vi "CRYFrequency Shift.vi"(6 "User Sampling Rate":dbl, 7 "Freq Sampling Mode":i32, 9 "Reference Frequency":dbl, 10 "Source Wave Name":string, 11 "Waveform In":T1={"Waveform"={"X0"=0.0, "dX"=0.0, "Y"=array[57657 elements]}, "X data"=1, "Y data"=0, "Y axis"=0, "X unit"="s", "Y unit"="", "Y dB ref"=1.0, "display Y"=TRUE, "display X"=FALSE, "Overload?"=FALSE, "Test Info"="", "Step No."=0, "Name"="", "protected"=FALSE, "Sqc history"=[], "Signal Channel ID"=0, "Plot Settings"={"Color"=0, "Interpolation"=0, "Point Style"=0, "Line Style"=0, "Point Color"=0, "Line Width"=0, "Bar Plot Style"=0, "Fill To"=0}, "AutoProtect"=FALSE} {"Y dB ref" format="%.1f"; "Y axis" items=["Log", "Lin"]; "Y data" items=["dB", "Lin"]; "X data" items=["dB", "Lin"]}) -> (2 "PlaybackSamplingRate":dbl, 3 "Wave Out":T1={"Waveform"={"X0"=0.0, "dX"=0.0, "Y"=[]}, "X data"=1, "Y data"=1, "Y axis"=1, "X unit"="s", "Y unit"="V", "Y dB ref"=1.0, "display Y"=TRUE, "display X"=TRUE, "Overload?"=FALSE, "Test Info"="", "Step No."=0, "Name"="", "protected"=FALSE, "Sqc history"=[], "Signal Channel ID"=0, "Plot Settings"={"Color"=0, "Interpolation"=0, "Point Style"=0, "Line Style"=0, "Point Color"=0, "Line Width"=0, "Bar Plot Style"=0, "Fill To"=0}, "AutoProtect"=FALSE} {"Y dB ref" format="%.1f"; "Y axis" items=["Log", "Lin"]; "Y data" items=["dB", "Lin"]; "X data" items=["dB", "Lin"]})   [LabVIEW 2013]
uses:
  Typedef Control/CRYWaveform Cluster.ctl
  <vilib>/Analysis/3filter.llb/Filter Passband Type.ctl
  <vilib>/Analysis/4window.llb/windowTd.ctl
  <vilib>/Analysis/2dsp.llb/Real FFT.vi
  <vilib>/Analysis/3filter.llb/FIR Windowed Filter (DBL).vi
  <vilib>/Analysis/NI_AALPro.lvlib
  <vilib>/Analysis/NI_AALBase.lvlib
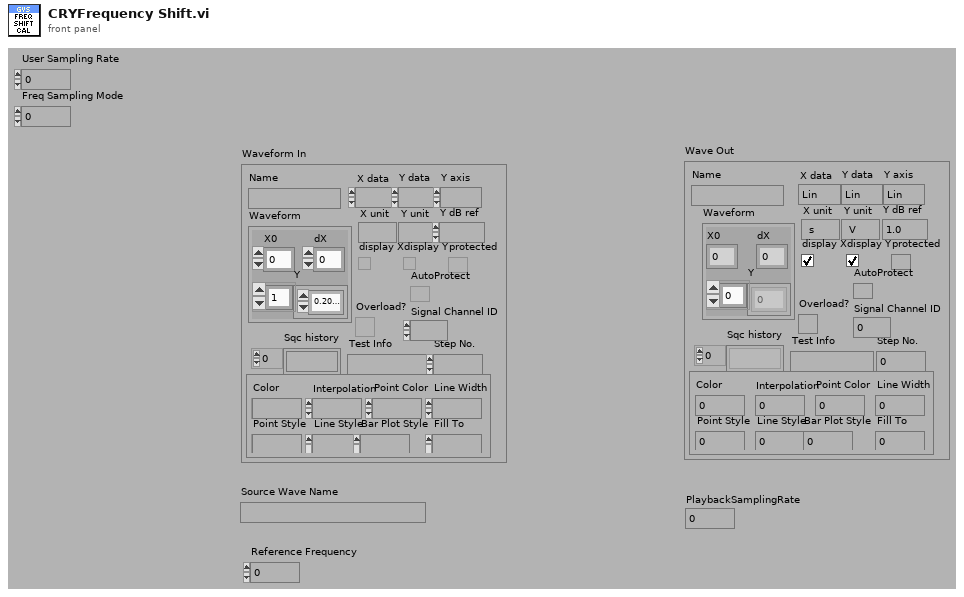
[diagram p1: front panel]
types:
  T1 = typedef "CRYWaveform Cluster.ctl" = cluster{"Waveform":cluster{"X0":dbl, "dX":dbl, "Y":sgl[]}, "X data":u16, "Y data":u16, "Y axis":u16, "X unit":string, "Y unit":string, "Y dB ref":dbl, "display Y":bool, "display X":bool, "Overload?":bool, "Test Info":string, "Step No.":i32, "Name":string, "protected":bool, "Sqc history":string[], "Signal Channel ID":i32, "Plot Settings":cluster{"Color":u32, "Interpolation":u8, "Point Style":u8, "Line Style":u8, "Point Color":u32, "Line Width":u8, "Bar Plot Style":u8, "Fill To":i16}, "AutoProtect":bool}
  T2 = typedef "NI_AALBase.lvlib/Filter Passband Type.ctl" = enum32{"Lowpass", "Highpass", "Bandpass", "Bandstop"}
  T3 = typedef "NI_AALPro.lvlib/windowTd.ctl" = u32
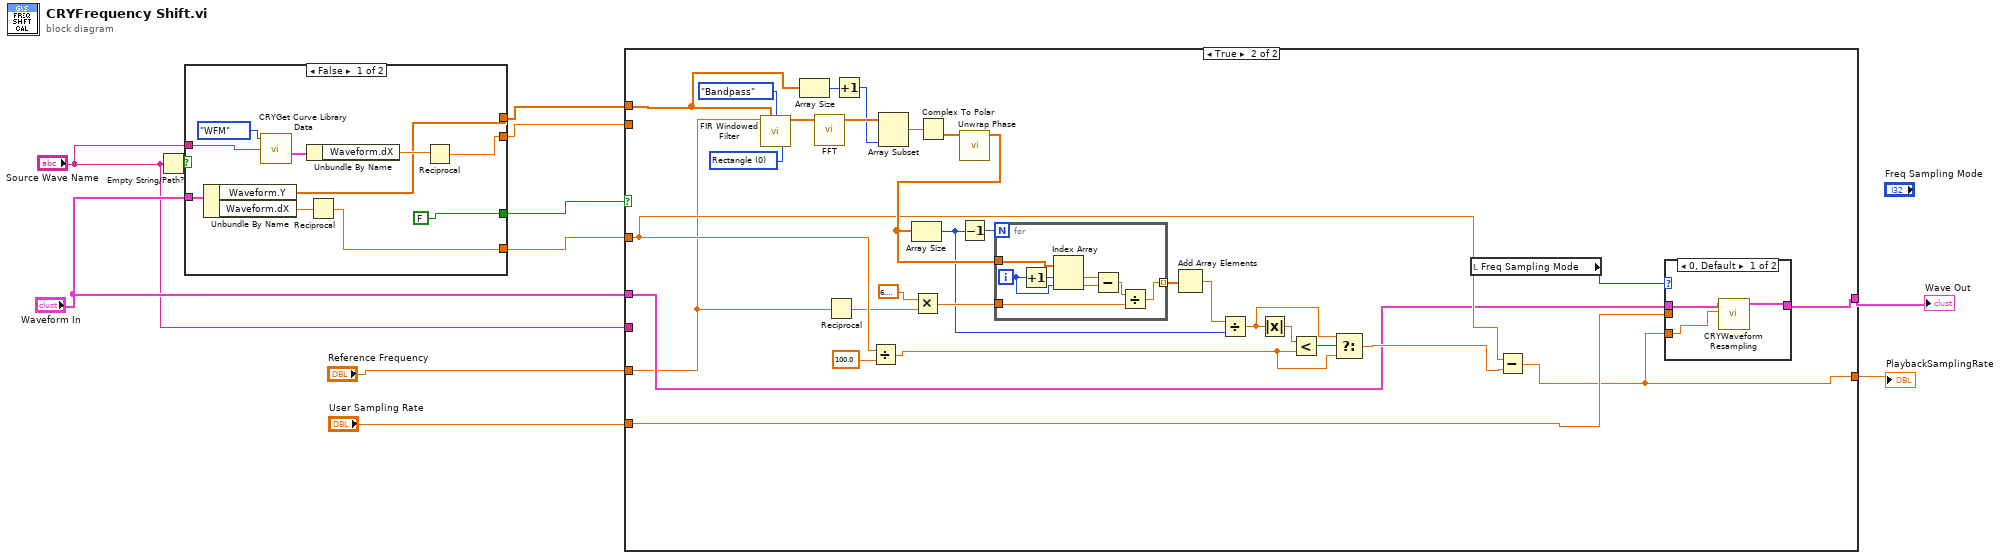
[diagram p0: block diagram]
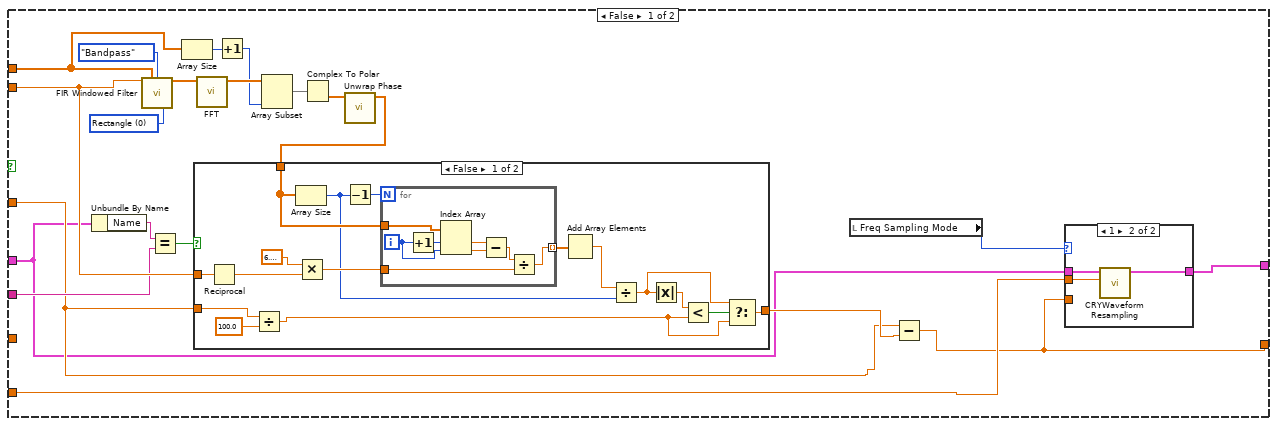
[diagram p2: hidden frame]
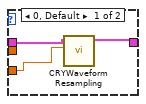
[diagram p3: hidden frame]
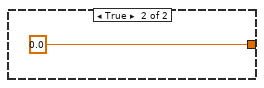
[diagram p4: hidden frame]
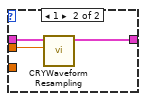
[diagram p5: hidden frame]
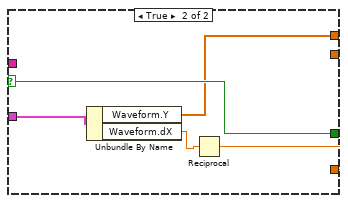
[diagram p6: hidden frame]
diagram:
  n1 = Empty String/Path?(string/path="Source Wave Name") -> (empty?=w11:bool)
  n2 = case shown="False" w11 {
    selector: w11 -> [_ w26]
    tunnel: [FALSE w26] -> w10
    tunnel: "Source Wave Name" -> [w19 _]
    tunnel: "Waveform In" -> [w18 w25]
    tunnel: [w13 w22] -> w1
    tunnel: [w14 _] -> w8
    tunnel: [w15 w23] -> w7
    frame False {
      n3 = Unbundle By Name(w18) -> ("Waveform.Y"=w13:sgl[], "Waveform.dX"=w17:dbl)
      n4 = call "CRYGet Curve Library Data.vi"("Type"=enum16{"Curves", "Values", "Results", "WFM"}."WFM", "Data Name"=w19) -> ("Wave"=w21:T1)  [unwired: 4 out]
      n5 = Unbundle By Name(w21) -> ("Waveform.dX"=w16:dbl)
      n6 = Reciprocal(x=w17) -> (1/x=w15:dbl)
      n7 = Reciprocal(x=w16) -> (1/x=w14:dbl)
    }
    frame True {
      n8 = Unbundle By Name(w25) -> ("Waveform.Y"=w22:sgl[], "Waveform.dX"=w24:dbl)
      n9 = Reciprocal(x=w24) -> (1/x=w23:dbl)
    }
  }
  n10 = case shown="True" w10 {
    tunnel: "Waveform In" -> [w30 w96]
    tunnel: [w35 w93] -> w2
    tunnel: [w28 w94] -> w3
    tunnel: w1 -> [w40 w98]
    tunnel: w8 -> [w37 _]
    tunnel: w7 -> [w31 w97]
    tunnel: "Source Wave Name" -> [w33 _]
    tunnel: "User Sampling Rate" -> [w29 w95]
    tunnel: "Reference Frequency" -> [_ w92]
    frame False {
      w42 = T3 0 items=["Rectangle"=0, "Hanning"=1, "Hamming"=2, "Blackman-Harris"=3, "Exact Blackman"=4, "Blackman"=5, "Flat Top"=6, "4 Term B-Harris "=7, "7 Term B-Harris"=8, "Low Sidelobe"=9, "Blackman Nuttall"=11, "Triangle"=30, "Bartlett-Hanning"=31, "Bohman"=32, "Parzen"=33, "Welch"=34, "Kaiser"=60, "Dolph-Chebyshev"=61, "Gaussian"=62] ("window")
      n11 = Unbundle By Name(w30) -> ("Name"=w34:string)
      n12 = call-poly <vilib>:"FIR Windowed Filter.vi"("sampling freq: fs"=w37, "X"=w40, "filter type"=Filter_Passband_Type."Bandpass", "window"=w42) -> ("Filtered X"=w44:dbl[])  [unwired: 10 in, 1 out]
      n13 = Equal?(x=w34, y=w33) -> (x = y?=w32:bool)
      n14 = Array Size(array=w40) -> (size(s)=w41:i32)
      n15 = call-poly <vilib>:"FFT.vi"("X"=w44) -> ("FFT {X}"=w46:cdb[])  [unwired: 9 in, 1 out]
      n16 = Increment(x=w41) -> (x+1=w39:i32)
      n17 = Array Subset(array=w46, length=w39) -> (w45:cdb[])  [unwired: 1 in]
      n18 = Complex To Polar(r * e^(i*theta)=w45) -> (theta=w47:dbl[])  [unwired: 1 out]
      n19 = call <vilib>:"Unwrap Phase.vi"("Phase"=w47) -> ("Unwrapped Phase"=w38:dbl[])  [unwired: 9 in, 1 out]
      n20 = case shown="False" w32 {
        tunnel: w38 -> [w66 _]
        tunnel: w37 -> [w65 _]
        tunnel: [w55 0.0] -> w36
        tunnel: w31 -> [w59 _]
        frame False {
          n21 = Reciprocal(x=w65) -> (1/x=w64:dbl)
          n22 = Divide(x=w59, y=100.0) -> (x/y=w56:dbl)
          n23 = Array Size(array=w66) -> (size(s)=w61:i32)
          n24 = Multiply(x=6.283185307179586, y=w64) -> (x*y=w67:dbl)
          n25 = Decrement(x=w61) -> (x-1=w69:i32)
          n26 = for {
            N: w69 -> [_]
            tunnel: w66 -> [w77]
            tunnel: [w70] -> w62 mode=indexing
            tunnel: w67 -> [w71]
            i -> [w75]
            n27 = Increment(x=w75) -> (x+1=w76:i32)
            n28 = Index Array(array=w77, index #1=w76, index #2=w75) -> (element #1=w74:dbl, element #2=w73:dbl)
            n29 = Subtract(x=w74, y=w73) -> (x-y=w72:dbl)
            n30 = Divide(x=w72, y=w71) -> (x/y=w70:dbl)
          }
          n31 = Add Array Elements(numeric array=w62) -> (sum=w63:dbl)
          n32 = Divide(x=w63, y=w61) -> (x/y=w54:dbl)
          n33 = Absolute Value(x=w54) -> (abs(x)=w57:dbl)
          n34 = Less?(x=w57, y=w56) -> (x < y?=w58:bool)
          n35 = Select(t=w54, s=w58, f=w56) -> (s? t:f=w55:dbl)
        }
        frame True {
        }
      }
      n36 = local read "Freq Sampling Mode"() -> (w27:i32)
      n37 = Subtract(x=w31, y=w36) -> (x-y=w28:dbl)
      n38 = case shown="1" w27 {
        tunnel: [w49 w53] -> w35
        tunnel: w30 -> [w50 w52]
        tunnel: w29 -> [_ w51]
        tunnel: w28 -> [w48 _]
        frame 0, Default {
          n39 = call "CRYWaveform Resampling.vi"("New Sampling Rate"=w48, "Wave"=w50) -> ("New Wave"=w49:T1)  [unwired: 9 in]
        }
        frame 1 {
          n40 = call "CRYWaveform Resampling.vi"("New Sampling Rate"=w51, "Wave"=w52) -> ("New Wave"=w53:T1)  [unwired: 9 in]
        }
      }
    }
    frame True {
      w103 = T3 0 items=["Rectangle"=0, "Hanning"=1, "Hamming"=2, "Blackman-Harris"=3, "Exact Blackman"=4, "Blackman"=5, "Flat Top"=6, "4 Term B-Harris "=7, "7 Term B-Harris"=8, "Low Sidelobe"=9, "Blackman Nuttall"=11, "Triangle"=30, "Bartlett-Hanning"=31, "Bohman"=32, "Parzen"=33, "Welch"=34, "Kaiser"=60, "Dolph-Chebyshev"=61, "Gaussian"=62] ("window")
      n41 = call-poly <vilib>:"FIR Windowed Filter.vi"("sampling freq: fs"=w92, "X"=w98, "filter type"=Filter_Passband_Type."Bandpass", "window"=w103) -> ("Filtered X"=w105:dbl[])  [unwired: 10 in, 1 out]
      n42 = Array Size(array=w98) -> (size(s)=w102:i32)
      n43 = call-poly <vilib>:"FFT.vi"("X"=w105) -> ("FFT {X}"=w107:cdb[])  [unwired: 9 in, 1 out]
      n44 = Reciprocal(x=w92) -> (1/x=w88:dbl)
      n45 = Increment(x=w102) -> (x+1=w101:i32)
      n46 = Divide(x=w97, y=100.0) -> (x/y=w81:dbl)
      n47 = Array Subset(array=w107, length=w101) -> (w106:cdb[])  [unwired: 1 in]
      n48 = Multiply(x=6.283185307179586, y=w88) -> (x*y=w89:dbl)
      n49 = Complex To Polar(r * e^(i*theta)=w106) -> (theta=w108:dbl[])  [unwired: 1 out]
      n50 = call <vilib>:"Unwrap Phase.vi"("Phase"=w108) -> ("Unwrapped Phase"=w100:dbl[])  [unwired: 9 in, 1 out]
      n51 = Array Size(array=w100) -> (size(s)=w85:i32)
      n52 = Decrement(x=w85) -> (x-1=w91:i32)
      n53 = for {
        N: w91 -> [_]
        tunnel: w100 -> [w116]
        tunnel: [w109] -> w86 mode=indexing
        tunnel: w89 -> [w110]
        i -> [w114]
        n54 = Increment(x=w114) -> (x+1=w115:i32)
        n55 = Index Array(array=w116, index #1=w115, index #2=w114) -> (element #1=w113:dbl, element #2=w112:dbl)
        n56 = Subtract(x=w113, y=w112) -> (x-y=w111:dbl)
        n57 = Divide(x=w111, y=w110) -> (x/y=w109:dbl)
      }
      n58 = Add Array Elements(numeric array=w86) -> (sum=w87:dbl)
      n59 = Divide(x=w87, y=w85) -> (x/y=w80:dbl)
      n60 = Absolute Value(x=w80) -> (abs(x)=w82:dbl)
      n61 = Less?(x=w82, y=w81) -> (x < y?=w83:bool)
      n62 = Select(t=w80, s=w83, f=w81) -> (s? t:f=w99:dbl)
      n63 = local read "Freq Sampling Mode"() -> (w79:i32)
      n64 = Subtract(x=w97, y=w99) -> (x-y=w94:dbl)
      n65 = case shown="0, Default" w79 {
        tunnel: [w118 w122] -> w93
        tunnel: w96 -> [w119 w121]
        tunnel: w95 -> [_ w120]
        tunnel: w94 -> [w117 _]
        frame 0, Default {
          n66 = call "CRYWaveform Resampling.vi"("New Sampling Rate"=w117, "Wave"=w119) -> ("New Wave"=w118:T1)  [unwired: 9 in]
        }
        frame 1 {
          n67 = call "CRYWaveform Resampling.vi"("New Sampling Rate"=w120, "Wave"=w121) -> ("New Wave"=w122:T1)  [unwired: 9 in]
        }
      }
    }
  }
  "Wave Out" <- w2
  "PlaybackSamplingRate" <- w3
